vi "Arduino Stepper Driver XY subVI moveSteps.vi"(8 "error in (no error)":errorcluster, 9 "input steps V":i32, 10 "input steps H":i32, 11 "VISA resource name":refnum<visa-resource-name>) -> (0 "error out":errorcluster, 3 "VISA resource name out":refnum<visa-resource-name>)   [LabVIEW 2013]
panel:
  out "read buffer":string
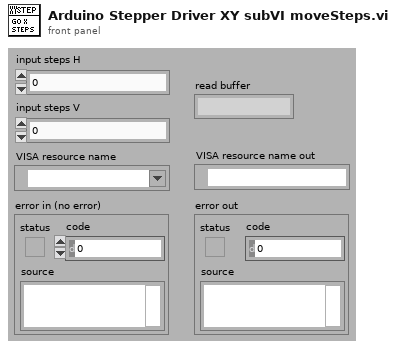
[diagram p1: front panel]
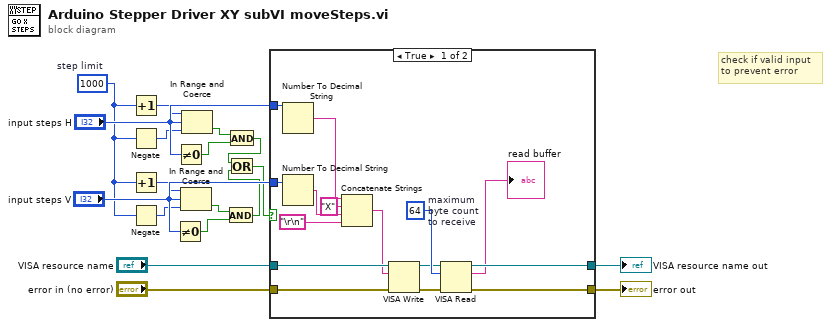
[diagram p0: block diagram]
diagram:
  w1 = 1000  # step limit
  # "check if valid input\nto prevent error"
  n1 = Increment(x=w1) -> (x+1=w3:i32)
  n2 = Negate(x=w1) -> (-x=w4:i32)
  n3 = Increment(x=w1) -> (x+1=w2:i32)
  n4 = Negate(x=w1) -> (-x=w5:i32)
  n5 = Not Equal To 0?(x="input steps V") -> (x != 0?=w16:bool)
  n6 = Not Equal To 0?(x="input steps H") -> (x != 0?=w10:bool)
  n7 = In Range and Coerce(upper limit=w2, x="input steps V", lower limit=w5) -> (In Range?=w17:bool)  [unwired: 1 out]
  n8 = In Range and Coerce(upper limit=w3, x="input steps H", lower limit=w4) -> (In Range?=w11:bool)  [unwired: 1 out]
  n9 = And(x=w17, y=w16) -> (x .and. y?=w7:bool)
  n10 = And(x=w11, y=w10) -> (x .and. y?=w8:bool)
  n11 = Or(x=w8, y=w7) -> (x .or. y?=w6:bool)
  n12 = case shown="True" w6 {
    tunnel: [w33 w35] -> w13
    tunnel: [w32 w34] -> w12
    tunnel: "VISA resource name" -> [w31 w35]
    tunnel: "error in (no error)" -> [w30 w34]
    tunnel: "input steps V" -> [w28 _]
    tunnel: "input steps H" -> [w23 _]
    frame True {
      w29 = u32 64  # maximum byte count to receive
      n13 = Number To Decimal String(number=w23) -> (decimal integer string=w20:string)  [unwired: 1 in]
      n14 = Number To Decimal String(number=w28) -> (decimal integer string=w22:string)  [unwired: 1 in]
      n15 = Concatenate Strings(w20, "X" ("string"), w22, "\r\n") -> (w26:string)
      n16 = VISA Write(VISA resource name=w31, write buffer=w26, error in (no error)=w30) -> (VISA resource name out=w25:refnum<visa-resource-name>, error out=w24:errorcluster)  [unwired: 1 out]
      n17 = VISA Read(VISA resource name=w25, byte count=w29, error in (no error)=w24) -> (VISA resource name out=w33:refnum<visa-resource-name>, read buffer=→"read buffer":string, error out=w32:errorcluster)  [unwired: 1 out]
    }
    frame False {
    }
  }
  "VISA resource name out" <- w13
  "error out" <- w12
